vi "repetitividade.vi"() -> ()   [LabVIEW 2011]
panel:
  out "Máximo desvio padrão":dbl format="%#.6g"
  out "Desvios Padrão":dbl[](array[numeric])
  in  "Menor valor do sinal":dbl
  in  "Maior valor do sinal":dbl
  out "Erro de Repetibilidade":dbl format="%#.6g"
  # "CÁLCULO DE REPETITIVIDADE"
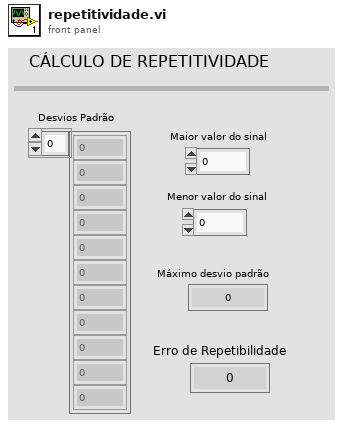
[diagram p1: front panel]
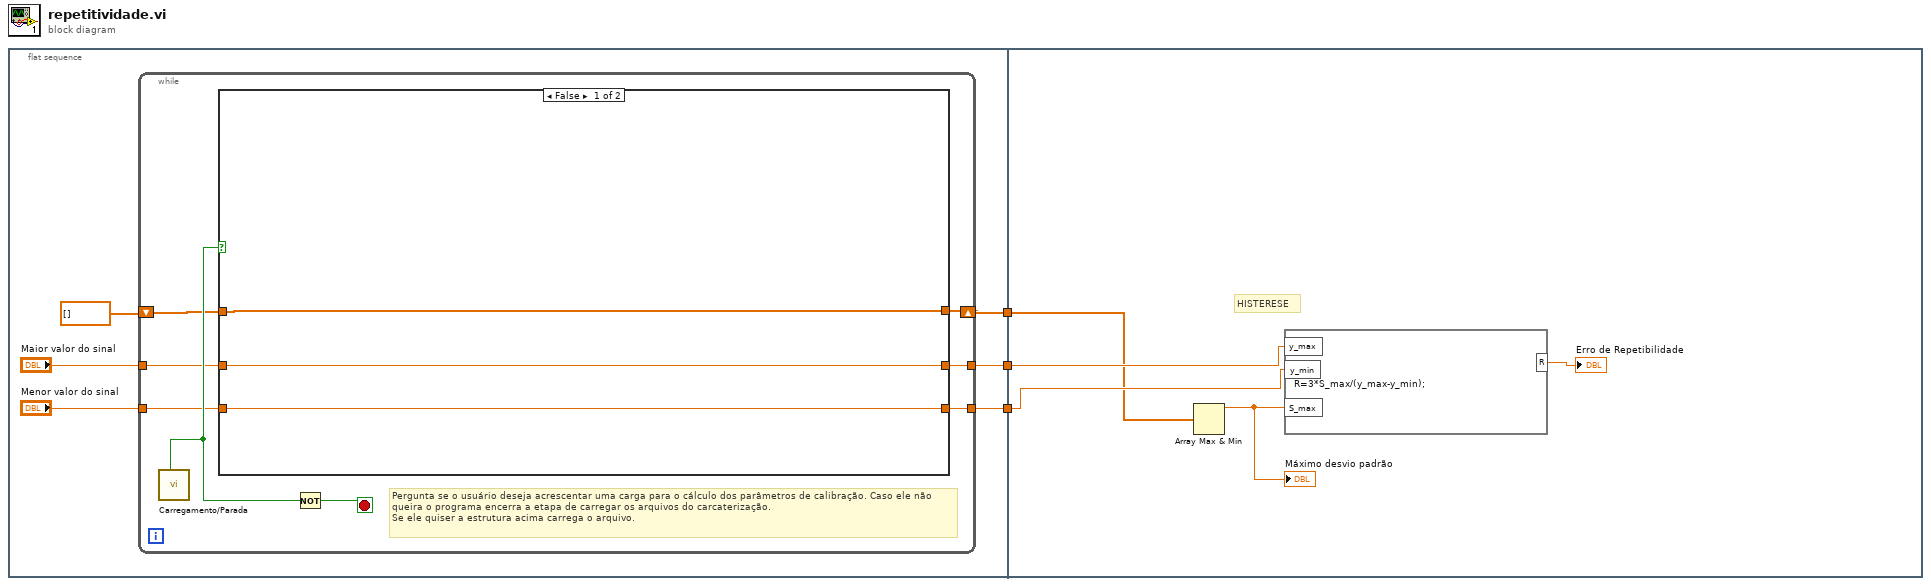
[diagram p0: block diagram]
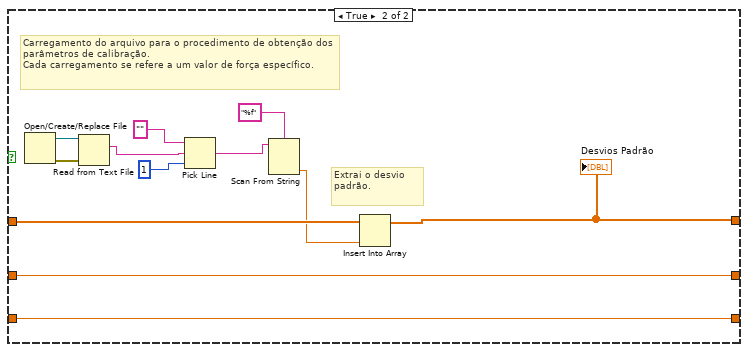
[diagram p2: hidden frame]
diagram:
  n1 = flat-sequence {
    tunnel: [w8] -> w3
    tunnel: [w5] -> w2
    tunnel: [w4] -> w1
    tunnel: w3 -> [w34]
    tunnel: w2 -> [w36]
    tunnel: w1 -> [w35]
    frame #0 {
      n2 = while {
        shift-right: [w14] -> w8
        shift-left: dbl[] [] ("array") -> [w15]
        tunnel: "Maior valor do sinal" -> [w13]
        tunnel: "Menor valor do sinal" -> [w12]
        tunnel: [w11] -> w5
        tunnel: [w10] -> w4
        stop <- w17 stop-if-true
        # "Pergunta se o usuário deseja acrescentar uma carga para o cálculo dos parâmetros de calibração. Caso ele não queira o programa encerra a etapa de carregar os arquivos do carcaterização.\nSe ele quiser a estrutura acima carrega o arquivo."
        n3 = call "Carregamento/Parada"() -> ("Carregar"=w16:bool)  [unwired: 18 in, 1 out]
        n4 = case shown="False" w16 {
          tunnel: w15 -> [w20 w30]
          tunnel: [w20 w29] -> w14
          tunnel: w13 -> [w19 w22]
          tunnel: w12 -> [w18 w21]
          tunnel: [w19 w22] -> w11
          tunnel: [w18 w21] -> w10
          frame False {
          }
          frame True {
            # "Carregamento do arquivo para o procedimento de obtenção dos parâmetros de calibração.\nCada carregamento se refere a um valor de força específico."
            # "Extrai o desvio padrão."
            n5 = Open/Create/Replace File() -> (refnum out=w32:refnum<file>, error out=w31:errorcluster)  [unwired: 6 in, 1 out]
            n6 = Read from Text File(file (use dialog)=w32, error in=w31) -> (text=w27:string)  [unwired: 2 in, 3 out]
            n7 = Pick Line(string ("")="", multi-line string=w27, line index=1) -> (output string=w25:string)
            n8 = Scan From String(format string="%f", input string=w25) -> (output 1=w23:dbl)  [unwired: 3 in, 3 out]
            n9 = Insert Into Array(array=w30, new element=w23) -> (w29:dbl[])  [unwired: 1 in]
            "Desvios Padrão" <- w29
          }
        }
        n10 = Not(x=w16) -> (.not. x?=w17:bool)
      }
    }
    frame #1 {
      # "HISTERESE"
      n11 = Array Max & Min(array=w34) -> (max value=w33:dbl)  [unwired: 3 out]
      "Máximo desvio padrão" <- w33
      n12 = formula code="R=3*S_max/(y_max-y_min);"("y_max"=w36, "S_max"=w33, "y_min"=w35) -> ("R"=→"Erro de Repetibilidade":dbl)
    }
  }
